vi "Check if Init APIs.vi"(0 "VIName":string) -> (4 "Instrument Driver Found?":bool, 6 "DAQ?":bool)   [LabVIEW 2021, in "Migrator.lvlib"]
uses:
  Migrator.lvlib
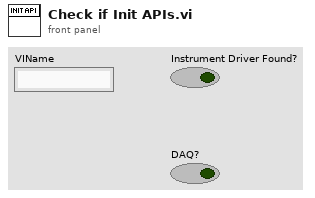
[diagram p1: front panel]
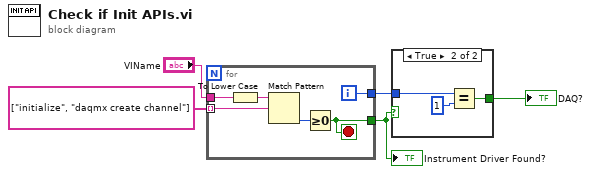
[diagram p0: block diagram]
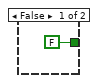
[diagram p2: hidden frame]
diagram:
  n1 = for {
    tunnel: "VIName" -> [w11]
    tunnel: [w6] -> w3
    tunnel: string[] ["initialize", "daqmx create channel"] ("regular expression") -> [w9] mode=indexing
    tunnel: [w7] -> w2
    i -> [w7]
    stop <- w6 stop-if-true
    n2 = To Lower Case(string=w11) -> (all lower case string=w10:string)
    n3 = Match Pattern(string=w10, regular expression=w9) -> (offset past match=w8:i32)  [unwired: 1 in, 3 out]
    n4 = Greater Or Equal To 0?(x=w8) -> (x >= 0?=w6:bool)
  }
  "Instrument Driver Found?" <- w3
  n5 = case shown="True" w3 {
    tunnel: w2 -> [_ w15]
    tunnel: [FALSE w13] -> w1
    frame False {
    }
    frame True {
      n6 = Equal?(x=w15, y=1) -> (x = y?=w13:bool)
    }
  }
  "DAQ?" <- w1
